vi "raw queue to image queue_grMD.vi"() -> ()   [LabVIEW 2012]
doc: "SciScan 1.2 160622"
uses:
  <vilib>/Utility/VariantDataType/Type.ctl
  GFG/GFGnumericGet.vi
  GFG/GFGbooleanGet.vi
  GFG/GFG library.lvlib
  <vilib>/Utility/VariantDataType/VariantType.lvlib
panel:
  out "error out 4":errorcluster
  out "error out 3":errorcluster
  out "error out 2":errorcluster
  out "# elements in raw queue":i32
  out "error out":errorcluster
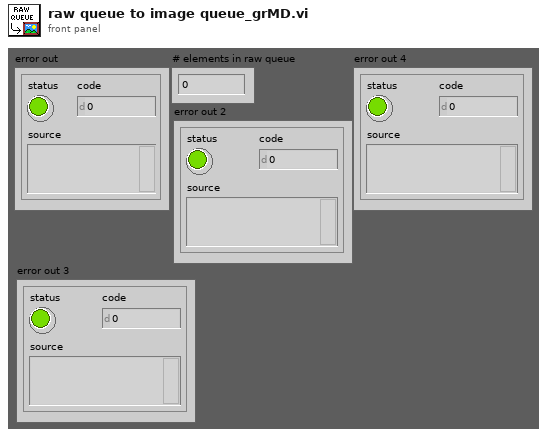
[diagram p1: front panel]
types:
  T1 = cluster{"NewVal":bool, "Event Registration Refnum":refnum<event-registration>}
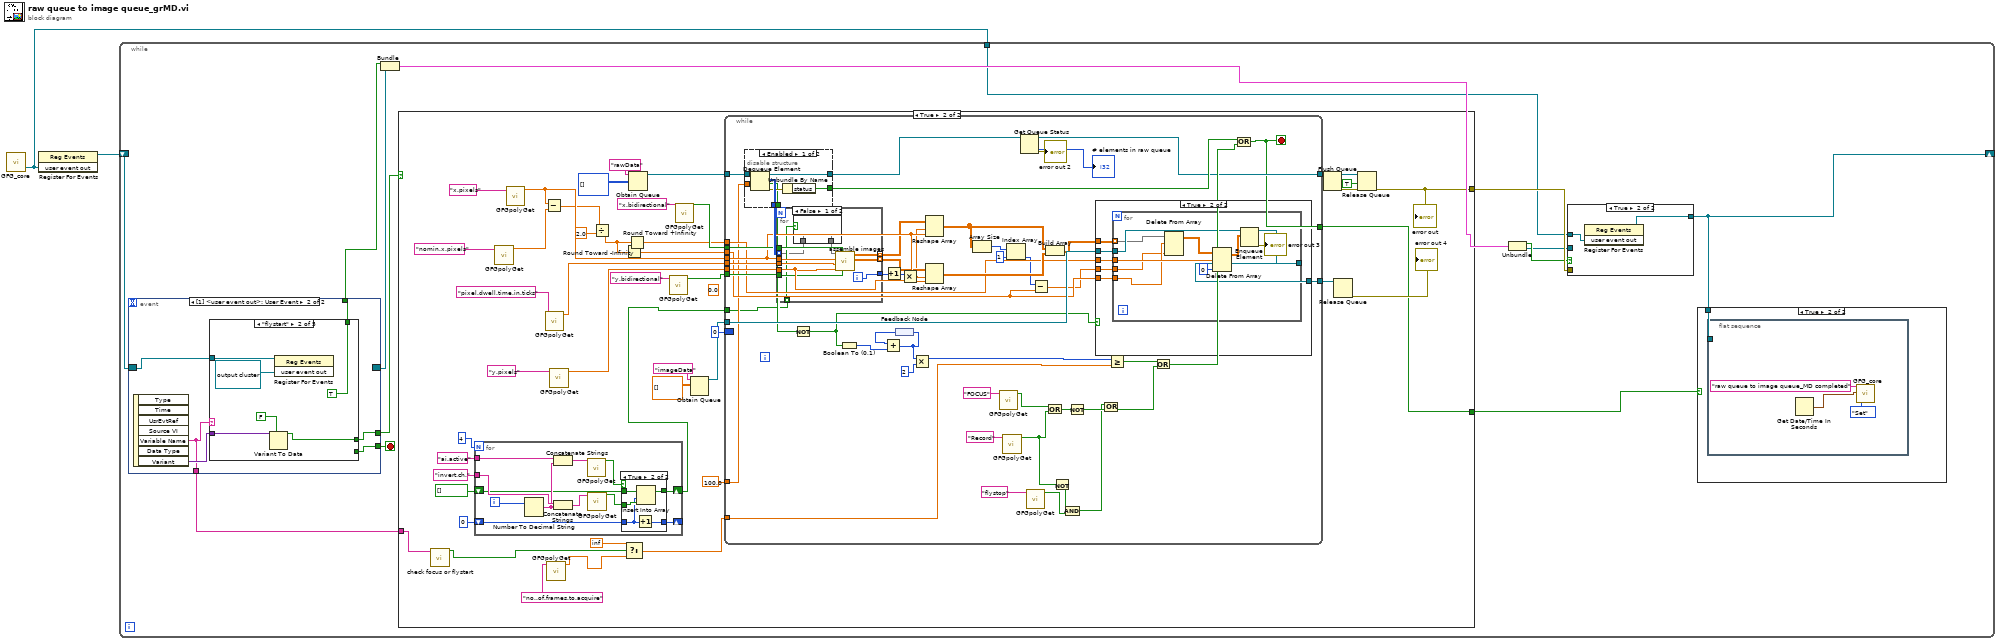
[diagram p0: block diagram]
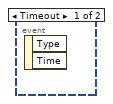
[diagram p4: hidden frame]
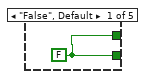
[diagram p5: hidden frame]
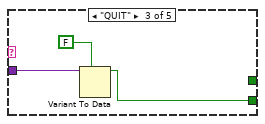
[diagram p6: hidden frame]
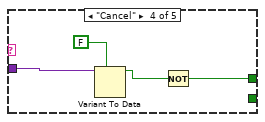
[diagram p7: hidden frame]
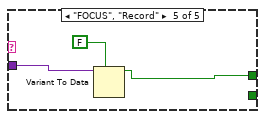
[diagram p8: hidden frame]
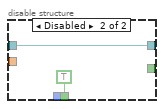
[diagram p11: hidden frame]
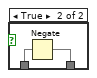
[diagram p13: hidden frame]
diagram:
  n1 = call "GFG_core.vi"() -> ("user event out"=w1:refnum<user-event>)  [unwired: 13 in, 6 out]
  n2 = register-events(w1) -> (reference out=w2:refnum<event-registration>)  [unwired: 2 in, 1 out]
  n3 = while {
    shift-right: [w4] -> _
    shift-left: w2 -> [w15]
    tunnel: w1 -> [w6]
    stop <- w14 stop-if-true
    n4 = event shown="[1] <user event out>: User Event" {
      selector: w15 -> [_ w25]
      dyn-events: [_ _] -> w11
      timeout: _ -> [_ _]
      tunnel: [_ w28] -> w13
      tunnel: [_ w27] -> w14
      tunnel: [_ w24] -> w12
      tunnel: [_ w23] -> w5
      event Timeout {
        n5 = event-data() -> ()  [unwired: 1 in, 2 out]
      }
      event User Event {
        n6 = event-data() -> ("Variable Name"=w23:string, "Variant"=w26:variant)  [unwired: 1 in, 5 out]
        n7 = case shown="\"flystart\"" w23 {
          tunnel: [w29 w33 _ w39 w43] -> w28
          tunnel: [w29 _ w36 _ _] -> w27
          tunnel: w26 -> [_ w34 w38 w41 w44]
          tunnel: w25 -> [_ w31 _ _ _]
          tunnel: [_ TRUE ("NewVal") _ _ _] -> w24
          frame "False", Default {
            w29 = FALSE ("NewVal")
          }
          frame "flystart" {
            n8 = Variant To Data(type=FALSE ("NewVal"), Variant=w34) -> (data=w33:bool)  [unwired: 1 in, 1 out]
            n9 = register-events(reference=w31, refnum<user-event> refnum ("user event out")) -> ()  [unwired: 1 in, 2 out]
          }
          frame "QUIT" {
            n10 = Variant To Data(type=FALSE ("NewVal"), Variant=w38) -> (data=w36:bool)  [unwired: 1 in, 1 out]
          }
          frame "Cancel" {
            n11 = Variant To Data(type=FALSE ("NewVal"), Variant=w41) -> (data=w40:bool)  [unwired: 1 in, 1 out]
            n12 = Not(x=w40) -> (.not. x?=w39:bool)
          }
          frame "FOCUS", "Record" {
            n13 = Variant To Data(type=FALSE ("NewVal"), Variant=w44) -> (data=w43:bool)  [unwired: 1 in, 1 out]
          }
        }
      }
    }
    n14 = Bundle("NewVal"=w12, "Event Registration Refnum"=w11) -> (w9:T1)  [unwired: 1 in]
    n15 = case shown="True" w13 {
      tunnel: [_ w62] -> w10
      tunnel: w5 -> [_ w58]
      tunnel: [_ w56] -> w3
      frame False {
      }
      frame True {
        (unwired) 0.0
        n16 = call "check focus or flystart.vi"("GFG variable name"=w58) -> ("Focus or flystart?"=w57:bool)  [unwired: 10 in]
        n17 = for {
          N: 4 -> [_]
          tunnel: "ai.active" ("Tag in") -> [w102]
          tunnel: "invert.ch." ("Tag in") -> [w99]
          shift-right: [w93] -> w47
          shift-left: bool[] [] ("Array") -> [w95]
          shift-right: [w92] -> _
          shift-left: 0 -> [w94]
          i -> [w91]
          n18 = Number To Decimal String(number=w91) -> (decimal integer string=w98:string)  [unwired: 1 in]
          n19 = Concatenate Strings(w102, w98) -> (w101:string)
          n20 = Concatenate Strings(w99, w98) -> (w100:string)
          n21 = call-poly "GFGpolyGet.vi"("Variable Name in"=w101) -> ("Boolean Value OUT"=w97:bool)  [unwired: 9 in, 1 out]
          n22 = call-poly "GFGpolyGet.vi"("Variable Name in"=w100) -> ("Boolean Value OUT"=w96:bool)  [unwired: 9 in, 1 out]
          n23 = case shown="True" w97 {
            tunnel: w96 -> [_ w108]
            tunnel: w95 -> [w103 w109]
            tunnel: w94 -> [w104 w106]
            tunnel: [w103 w107] -> w93
            tunnel: [w104 w105] -> w92
            frame False {
            }
            frame True {
              n24 = Increment(x=w106) -> (x+1=w105:i32)
              n25 = Insert Into Array(array=w109, index=w106, new element=w108) -> (w107:bool[])
            }
          }
        }
        n26 = call-poly "GFGpolyGet.vi"("Variable Name in"="nomin.x.pixels" ("Tag in")) -> ("Numeric"=w70:dbl)  [unwired: 8 in, 2 out]
        n27 = call-poly "GFGpolyGet.vi"("Variable Name in"="x.pixels" ("Tag in")) -> ("Numeric"=w69:dbl)  [unwired: 8 in, 2 out]
        n28 = Subtract(x=w69, y=w70) -> (x-y=w68:dbl)
        n29 = call-poly "GFGpolyGet.vi"("Variable Name in"="pixel.dwell.time.in.ticks" ("Tag in")) -> ("Numeric"=w80:dbl)  [unwired: 8 in, 2 out]
        n30 = call-poly "GFGpolyGet.vi"("Variable Name in"="no..of.frames.to.acquire" ("Tag in")) -> ("Numeric"=w54:dbl)  [unwired: 8 in, 2 out]
        n31 = call-poly "GFGpolyGet.vi"("Variable Name in"="y.pixels" ("Tag in")) -> ("Numeric"=w73:dbl)  [unwired: 8 in, 2 out]
        n32 = Divide(x=w68, y=2.0) -> (x/y=w65:dbl)
        n33 = Round Toward -Infinity(1:w65) -> (0:w64:dbl)
        n34 = Select(t=inf, s=w57, f=w54) -> (s? t:f=w59:dbl)
        n35 = Round Toward +Infinity(x=w65) -> (ceil(x): smallest int >= x=w66:dbl)
        n36 = Obtain Queue(name (unnamed)="rawData", element data type=i16[][] [] ("-x")) -> (queue out=w85:refnum<queue>)  [unwired: 3 in, 2 out]
        n37 = call-poly "GFGpolyGet.vi"("Variable Name in"="y.bidirectional") -> ("Boolean Value OUT"=w77:bool)  [unwired: 9 in, 1 out]
        n38 = call-poly "GFGpolyGet.vi"("Variable Name in"="x.bidirectional") -> ("Boolean Value OUT"=w75:bool)  [unwired: 9 in, 1 out]
        n39 = Obtain Queue(name (unnamed)="imageData", element data type=dbl[][] [] ("y backward image")) -> (queue out=w87:refnum<queue>)  [unwired: 3 in, 2 out]
        n40 = while {
          tunnel: w85 -> [w150]
          tunnel: [w143] -> w83
          tunnel: w87 -> [w161]
          tunnel: [w160] -> w86
          tunnel: w69 -> [w154]
          tunnel: w73 -> [w159]
          tunnel: w80 -> [w158]
          tunnel: w77 -> [w156]
          tunnel: w75 -> [w155]
          tunnel: w59 -> [w152]
          tunnel: 100.0 -> [w117]
          tunnel: w66 -> [w134]
          tunnel: w64 -> [w129]
          tunnel: [w125] -> w56
          border: i16 0 -> [_]
          tunnel: w47 -> [w110]
          stop <- w125 stop-if-true
          n41 = disable-structure shown="Enabled" {
            disable-tunnel: [w168 _] -> w157
            disable-tunnel: [w167 _] -> w153
            disable-tunnel: w150 -> [w165 w170]
            disable-tunnel: [w164 w170] -> w144
            disable-tunnel: [w163 TRUE ("timed out?")] -> w118
            disable-tunnel: w117 -> [w162 _]
            frame Enabled {
              n42 = Dequeue Element(queue=w165, timeout in ms (-1)=w162) -> (queue out=w164:refnum<queue>, element=w168:i16[][], timed out?=w163:bool, error out=w166:errorcluster)  [unwired: 1 in]
              n43 = Unbundle By Name(w166) -> ("status"=w167:bool)
            }
            frame Disabled {
            }
          }
          n44 = for {
            tunnel: w157 -> [w189] mode=indexing
            tunnel: w158 -> [w197]
            tunnel: w154 -> [w196]
            tunnel: w159 -> [w198]
            tunnel: [w195] -> w140 mode=indexing
            tunnel: [w194] -> w139 mode=indexing
            tunnel: w156 -> [w192]
            tunnel: w155 -> [w193]
            tunnel: [w191] -> w136
            tunnel: w110 -> [w190] mode=indexing
            i -> [w191]
            n45 = case shown="False" w190 {
              tunnel: [w199 w200] -> w188
              tunnel: w189 -> [w199 w201]
              frame False {
              }
              frame True {
                n46 = Negate(x=w201) -> (-x=w200:i16[])
              }
            }
            n47 = call "assemble images.vi"("bidi_y"=w192, "bidi_x"=w193, "y pixels"=w198, "bin factor"=w197, "x pixels"=w196, "raw data in (negative 11 bit data)"=w188) -> ("second image"=w194:dbl[][], "first image"=w195:dbl[][])  [unwired: 4 in]
          }
          n48 = Not(x=w118) -> (.not. x?=w114:bool)
          n49 = Boolean To (0,1)(Boolean=w114) -> (0, 1=w113:i16)
          n50 = Increment(x=w136) -> (x+1=w135:i32)
          n51 = feedback #1() -> (w112:i16)
          n52 = Add(x=w112, y=w113) -> (x+y=w111:i16)
          n53 = feedback-in #1(w111) -> ()
          n54 = Multiply(x=w135, y=w159) -> (x*y=w138:dbl)
          n55 = Multiply(x=w111, y=2) -> (x*y=w116:i32)
          n56 = Reshape Array(w140, w138, w154) -> (w133:dbl[][])
          n57 = Reshape Array(w139, w138, w154) -> (w137:dbl[][])
          n58 = Array Size(array=w133) -> (size(s)=w132:i32[])
          n59 = call-poly "GFGpolyGet.vi"("Variable Name in"="FOCUS") -> ("Boolean Value OUT"=w147:bool)  [unwired: 9 in, 1 out]
          n60 = call-poly "GFGpolyGet.vi"("Variable Name in"="Record") -> ("Boolean Value OUT"=w121:bool)  [unwired: 9 in, 1 out]
          n61 = Index Array(array=w132, index=1) -> (element=w130:i32)
          n62 = Get Queue Status(queue=w144) -> (queue out=w143:refnum<queue>, error out=→"error out 2":errorcluster, # elements in queue=→"# elements in raw queue":i32)  [unwired: 2 in, 5 out]
          n63 = call-poly "GFGpolyGet.vi"("Variable Name in"="flystop") -> ("Boolean Value OUT"=w122:bool)  [unwired: 9 in, 1 out]
          n64 = Subtract(x=w130, y=w129) -> (x-y=w128:dbl)
          n65 = Build Array(w133, w137) -> (w141:dbl[][][])
          n66 = Or(x=w147, y=w121) -> (x .or. y?=w145:bool)
          n67 = Not(x=w121) -> (.not. x?=w123:bool)
          n68 = And(x=w123, y=w122) -> (x .and. y?=w119:bool)
          n69 = Not(x=w145) -> (.not. x?=w126:bool)
          n70 = case shown="True" w114 {
            tunnel: w161 -> [w171 w177]
            tunnel: [w171 w176] -> w160
            tunnel: w141 -> [_ w175]
            tunnel: w134 -> [_ w174]
            tunnel: w129 -> [_ w173]
            tunnel: w128 -> [_ w172]
            frame False {
            }
            frame True {
              n71 = for {
                tunnel: w175 -> [w180] mode=indexing
                tunnel: w177 -> [w187]
                tunnel: [w186] -> w176
                tunnel: w174 -> [w185]
                tunnel: w173 -> [w183]
                tunnel: w172 -> [w182]
                n72 = Delete From Array(array=w180, length=w183, index (col)=w182) -> (array with subset deleted=w181:dbl[][])  [unwired: 1 in, 1 out]
                n73 = Delete From Array(array=w181, length=w185, index (col)=0 ("disabled index (col)")) -> (array with subset deleted=w179:dbl[][])  [unwired: 1 in, 1 out]
                n74 = Enqueue Element(queue=w187, element=w179) -> (queue out=w186:refnum<queue>, error out=→"error out 3":errorcluster)  [unwired: 2 in, 1 out]
              }
            }
          }
          n75 = Or(x=w119, y=w126) -> (x .or. y?=w120:bool)
          n76 = Greater Or Equal?(x=w116, y=w152) -> (x >= y?=w151:bool)
          n77 = Or(x=w151, y=w120) -> (x .or. y?=w146:bool)
          n78 = Or(x=w153, y=w146) -> (x .or. y?=w125:bool)
        }
        n79 = Flush Queue(queue=w83) -> (queue out=w82:refnum<queue>, error out=w72:errorcluster)  [unwired: 1 in, 1 out]
        n80 = Release Queue(queue=w86) -> (error out=→"error out 4":errorcluster)  [unwired: 2 in, 2 out]
        n81 = Release Queue(queue=w82, force destroy? (F)=TRUE, error in (no error)=w72) -> (error out=w62:errorcluster)  [unwired: 2 out]
        "error out" <- w62
      }
    }
    n82 = Unbundle(w9) -> ("NewVal"=w8:bool, "Event Registration Refnum"=w7:refnum<event-registration>)
    n83 = case shown="True" w8 {
      tunnel: [w20 w22] -> w4
      tunnel: w10 -> [_ _]
      tunnel: w7 -> [w20 _]
      tunnel: w6 -> [_ w21]
      frame False {
      }
      frame True {
        n84 = register-events(w21) -> (reference out=w22:refnum<event-registration>)  [unwired: 2 in, 1 out]
      }
    }
    n85 = case shown="True" w3 {
      tunnel: w4 -> [_ w16]
      frame False {
      }
      frame True {
        n86 = flat-sequence {
          tunnel: w16 -> [_]
          frame #0 {
            n87 = Get Date/Time In Seconds() -> (seconds since 1Jan1904=w17:timestamp)
            n88 = call "GFG_core.vi"("Variable Name in"="raw queue to image queue_MD completed", "Variant in"=w17, "Action"=enum16{"Init", "Set", "Get"}."Set") -> ()  [unwired: 10 in, 7 out]
          }
        }
      }
    }
  }
